vi "Get Child Window Bounds.vi"(8 "error in (no error)":errorcluster, 11 "Child Hwnd":u32) -> (0 "error out":errorcluster, 3 "Bounds":T1)   [LabVIEW 2016, in "LV MDI.lvclass"]
doc: "Retrieves the dimensions of the bounding rectangle of the specified child swindow."
uses:
  LV MDI.lvclass
  protected/Postion.ctl
  user32.dll
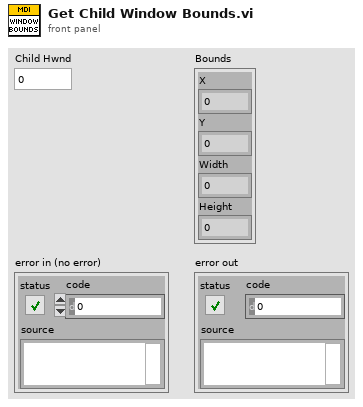
[diagram p1: front panel]
types:
  T1 = typedef "Postion.ctl" = cluster{"X":i32, "Y":i32, "Width":i32, "Height":i32}
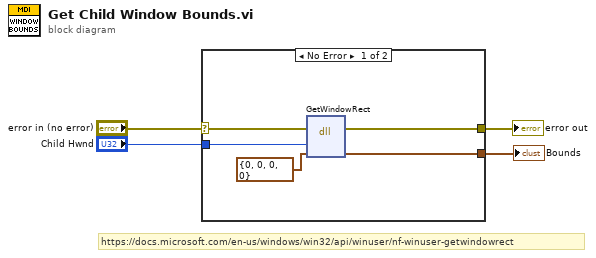
[diagram p0: block diagram]
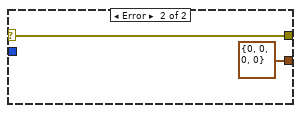
[diagram p2: hidden frame]
diagram:
  # "https://docs.microsoft.com/en-us/windows/win32/api/winuser/nf-winuser-getwindowrect"
  n1 = case shown="No Error" "error in (no error)" {
    selector: "error in (no error)" -> [w8 w11]
    tunnel: [w9 T1 {"X"=0, "Y"=0, "Width"=0, "Height"=0} ("lpRect")] -> w4
    tunnel: [w7 w11] -> w2
    tunnel: "Child Hwnd" -> [w6 _]
    frame No Error {
      n2 = dll-call lib="user32.dll" fn="GetWindowRect"(error in=w8, "Hwnd"=w6, "lpRect"=T1 {"X"=0, "Y"=0, "Width"=0, "Height"=0} ("Position")) -> (error out=w7:errorcluster, "lpRect"=w9:T1)  [unwired: 4 in, 1 out]
    }
    frame Error {
    }
  }
  "Bounds" <- w4
  "error out" <- w2
